vi "RefreshList.vi"(8 "error in (no error)":errorcluster, 11 "DAQ_Module in":refnum<class "DAQ_Module.lvclass">) -> (0 "error out":errorcluster, 3 "DAQ_Module out":refnum<class "DAQ_Module.lvclass">)   [LabVIEW 2025, in "DAQ_Module.lvlib" / "DAQ_Module.lvclass"]
uses:
  DAQ_Module.lvclass
  DAQ_Module.lvclass/DAQ_Module.ctl
  DAQ_Abstr/Task_Abstr/Task_Abstr Messages/GetTaskStatus Msg/GetTaskStatus Msg.lvclass/GetTaskStatus Msg.ctl
  <vilib>/ActorFramework/Message Enqueuer/Message Enqueuer.lvclass/Message Enqueuer.ctl
  <vilib>/ActorFramework/Message Enqueuer/Enqueue.vi
  DAQ_Abstr/Task_Abstr/Task_Abstr Messages/GetTaskStatus Msg/GetTaskStatus Msg.lvclass
  <vilib>/ActorFramework/Message Priority Queue/Priority Enqueue.vi
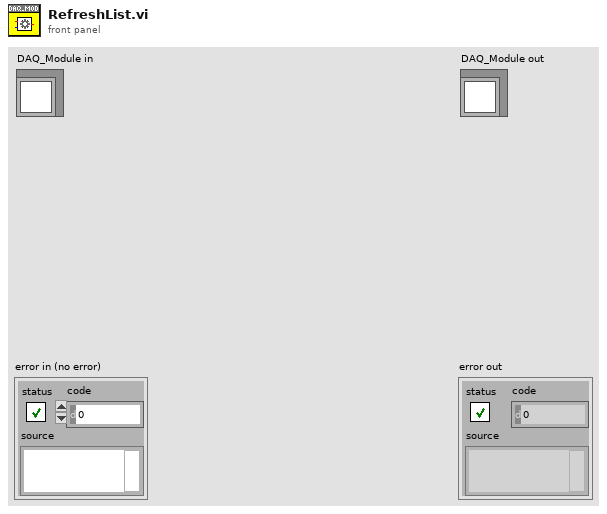
[diagram p1: front panel]
types:
  T1 = map{string, refnum<class "Message Enqueuer.lvclass">}
  T2 = typedef "DAQ_Module.lvlib/DAQ_Module.lvclass/DAQ_Task_Config.ctl" = cluster{"Drive":T3, "TaskType":T4, "PhysicalChannels":string, "SampleRateConfiguration":T5, "ChannelConfig":map{string, cluster{"Name":string, "Config":string}}, "Enable":bool, "Original":bool}
  T3 = typedef "DAQ_Module.lvlib/DAQ_Module.lvclass/DAQ_HW_Type.ctl" = enum16{"NI_DAQmx", "Simulated_DAQ"}
  T4 = typedef "DAQ_Module.lvlib/DAQ_Module.lvclass/DAQ_Task_Type.ctl" = enum16{"AI", "Linear", "Angular", "AO"}
  T5 = typedef "DAQ_Module.lvlib/DAQ_Module.lvclass/DAQ_SampleRateConfig.ctl" = cluster{"SampleRate":dbl, "SamplesPerChannel":u32, "SamplesPerRead":i32, "SampleMode":i32, "Clock Source":string}
  T6 = cluster{"Acessors:Running":bool, "Acessors:Record":bool, "Acessors:RecordLabel":string, "Acessors:TaskConfig":T2, "TDMS_Path":path}
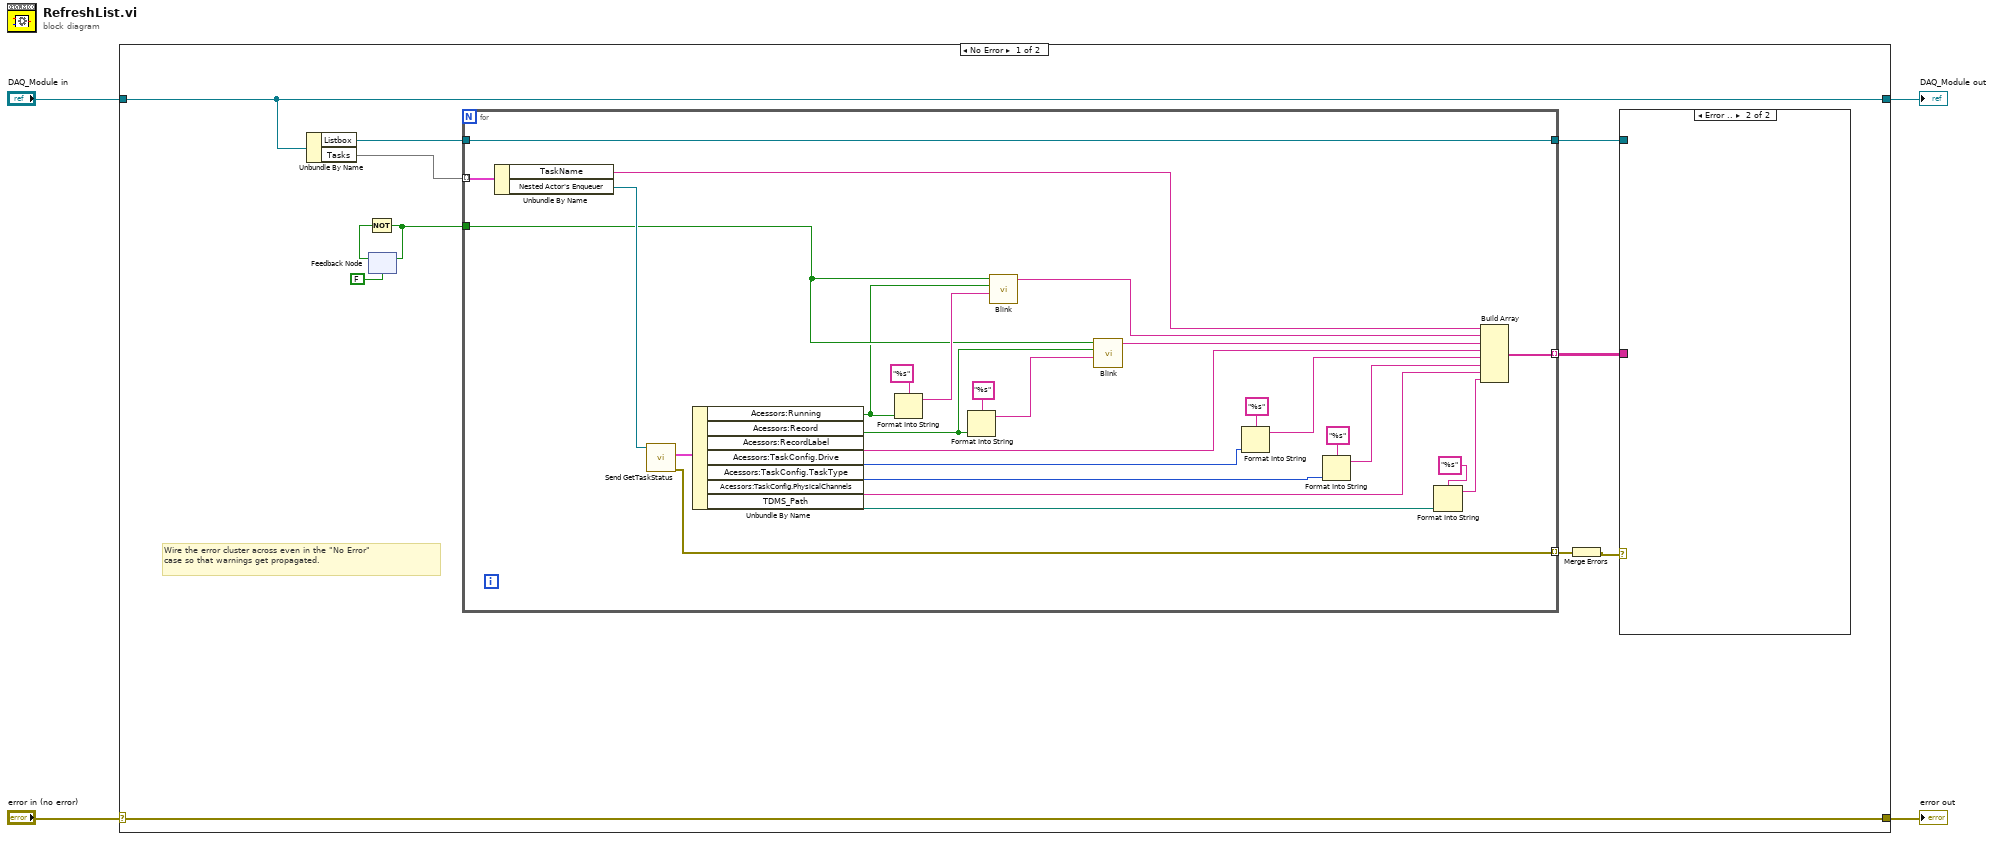
[diagram p0: block diagram]
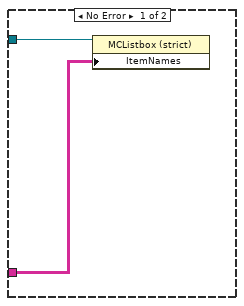
[diagram p2: hidden frame]
diagram:
  n1 = case shown="No Error" "error in (no error)" {
    selector: "error in (no error)" -> [w15 w46]
    tunnel: [w15 w46] -> w3
    tunnel: [w14 w45] -> w1
    tunnel: "DAQ_Module in" -> [w14 w45]
    frame No Error {
      # "Wire the error cluster across even in the \"No Error\"\ncase so that warnings get propagated."
      n2 = Unbundle By Name(w14) -> ("Listbox"=w11:refnum<vi>, "Tasks"=w13:T1)
      n3 = feedback #1(FALSE) -> (w9:bool)
      n4 = Not(x=w9) -> (.not. x?=w7:bool)
      n5 = feedback-in #1(w7) -> ()
      n6 = for {
        tunnel: w13 -> [w44] mode=indexing
        tunnel: [w30] -> w12 mode=indexing
        tunnel: w11 -> [w26]
        tunnel: [w26] -> w10
        tunnel: w7 -> [w22]
        tunnel: [w18] -> w6 mode=indexing
        n7 = Unbundle By Name(w44) -> ("TaskName"=w41:string, "Nested Actor's Enqueuer"=w43:refnum<class "Message Enqueuer.lvclass">)
        n8 = call "Send GetTaskStatus.vi"("Message Enqueuer"=w43) -> ("error out"=w18:errorcluster, "TaskStatus"=w42:T6)  [unwired: 8 in, 1 out]
        n9 = Unbundle By Name(w42) -> ("Acessors:Running"=w21:bool, "Acessors:Record"=w19:bool, "Acessors:RecordLabel"=w38:string, "Acessors:TaskConfig.Drive"=w36:T3, "Acessors:TaskConfig.TaskType"=w33:T4, "Acessors:TaskConfig.PhysicalChannels"=w31:string, "TDMS_Path"=w29:path)
        n10 = Format Into String(format string="%s", w21) -> (resulting string=w25:string)  [unwired: 2 in, 1 out]
        n11 = Format Into String(format string="%s", w19) -> (resulting string=w23:string)  [unwired: 2 in, 1 out]
        n12 = call "Blink.vi"("String"=w25, "Acessors:Running"=w21, "Checkbox"=w22) -> ("f"=w24:string)  [unwired: 8 in]
        n13 = call "Blink.vi"("String"=w23, "Acessors:Running"=w19, "Checkbox"=w22) -> ("f"=w20:string)  [unwired: 8 in]
        n14 = Format Into String(format string="%s", w36) -> (resulting string=w35:string)  [unwired: 2 in, 1 out]
        n15 = Format Into String(format string="%s", w33) -> (resulting string=w32:string)  [unwired: 2 in, 1 out]
        n16 = Format Into String(format string="%s", w29) -> (resulting string=w27:string)  [unwired: 2 in, 1 out]
        n17 = Build Array(w41, w24, w20, w38, w35, w32, w31, w27) -> (w30:string[])
      }
      n18 = Merge Errors(w6) -> (w5:errorcluster)
      n19 = case shown="Error .." w5 {
        tunnel: w12 -> [w17 _]
        tunnel: w10 -> [w16 _]
        frame No Error {
          n20 = property class="MCListbox (strict)"(reference=w16, "ItemNames"=w17) -> ()  [unwired: 1 in, 2 out]
        }
        frame Error {
        }
      }
    }
    frame Error {
    }
  }
  "error out" <- w3
  "DAQ_Module out" <- w1
